vi "WSVCAP SHL Host LL RFFE Build and Parse Data.vi"(0 "Data Out":string, 1 "Data Out (Cycle Commands)":string[](array[string]), 2 "Post Command Delay":dbl[](array[numeric]) format="%#.0p s", 7 "Clock Rate (Hz) (Cycle Only)":dbl=50000.0, 9 "RFFE Data In [U8]":u8[][](array[numeric]) format="%02x", 12 "Simulate FPGA (Cycle Only)":bool, 13 "DUT Mask (All)":bool[](array[boolean])=[TRUE, TRUE, TRUE, TRUE, TRUE, TRUE, TRUE, TRUE, TRUE, TRUE, TRUE, TRUE, TRUE, TRUE, TRUE, TRUE, TRUE, TRUE, TRUE, TRUE, TRUE, TRUE, TRUE, TRUE, TRUE, TRUE, TRUE, TRUE, TRUE, TRUE, TRUE, TRUE, TRUE, TRUE, TRUE, TRUE]) -> (4 "RFFE Data Out [U8]":u8[][](array[numeric]) format="%02x", 6 "CMD Lengths (Bits)":u8[](array[numeric]), 8 "CMD Delays (Ticks)":u32[](array[numeric]), 10 "RFFE Data In":string[](array[string]))   [LabVIEW 2012]
panel:
  # "DUT 01"
  # "DUT 02"
  # "DUT 03"
  # "DUT 04"
  # "DUT 05"
  # "DUT 06"
  # "DUT 07"
  # "DUT 08"
  # "DUT 09"
  # "DUT 10"
  # "DUT 11"
  # "DUT 12"
  # "DUT 13"
  # "DUT 14"
  # "DUT 15"
  # "DUT 16"
  # "DUT 17"
  # "DUT 18"
  # "DUT 19"
  # "DUT 20"
  # "DUT 21"
  # "DUT 22"
  # "DUT 23"
  # "DUT 24"
  # "DUT 25"
  # "DUT 26"
  # "DUT 27"
  # "DUT 28"
  # "DUT 29"
  # "DUT 30"
  # "DUT 31"
  # "DUT 32"
  # "DUT 33"
  # "DUT 34"
  # "DUT 35"
  # "DUT 36"
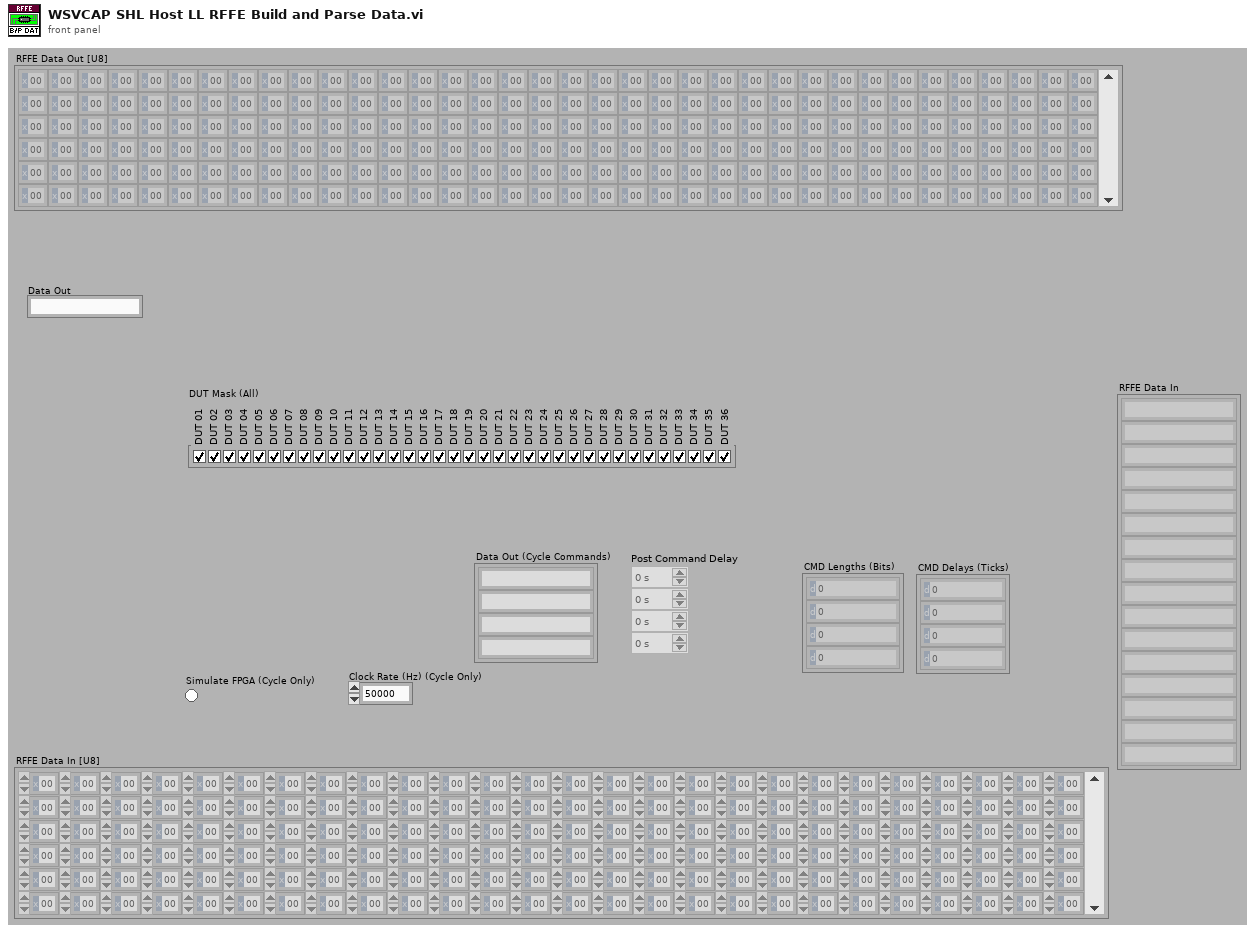
[diagram p1: front panel]
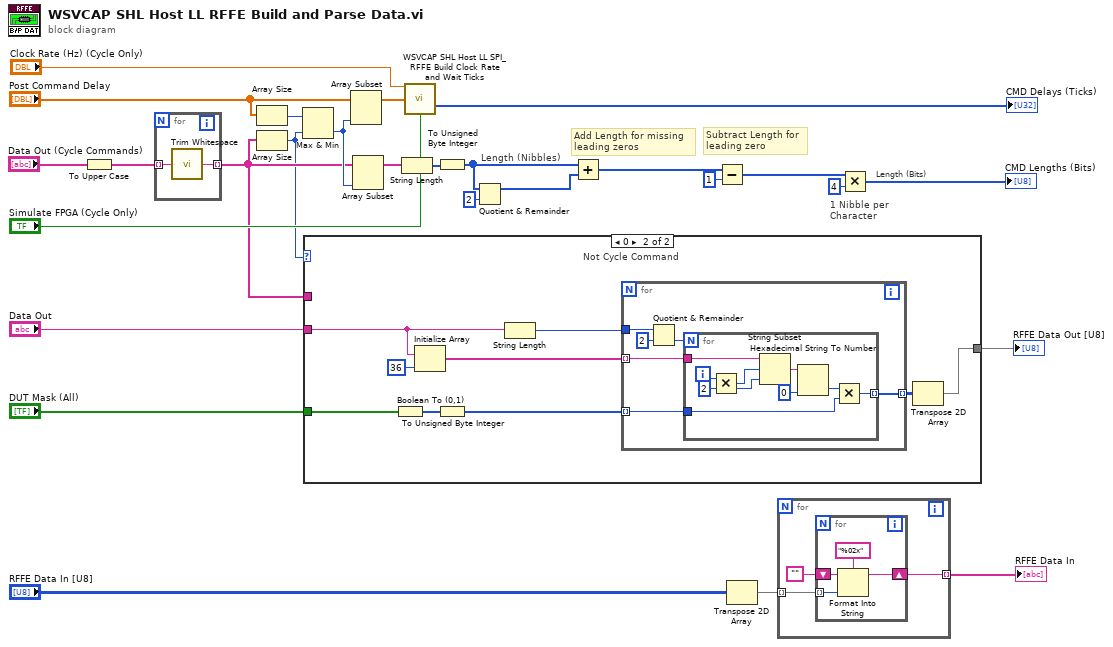
[diagram p0: block diagram]
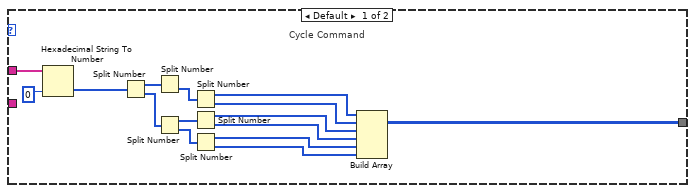
[diagram p2: hidden frame]
diagram:
  # "Subtract Length for\nleading zero"
  # "Add Length for missing\nleading zeros"
  # "Length (Bits)"
  # "Length (Nibbles)"
  # "1 Nibble per Character"
  n1 = To Upper Case(1:"Data Out (Cycle Commands)") -> (0:w1:string[])
  n2 = for {
    tunnel: w1 -> [w29] mode=indexing
    tunnel: [w28] -> w12 mode=indexing
    n3 = call <vilib>:"Trim Whitespace.vi"("string"=w29) -> ("trimmed string"=w28:string)  [unwired: 1 in]
  }
  n4 = Array Size(array="Post Command Delay") -> (size(s)=w21:i32)
  n5 = Array Size(array=w12) -> (size(s)=w11:i32)
  n6 = Max & Min(x=w21, y=w11) -> (min(x,y)=w18:i32)  [unwired: 1 out]
  n7 = case shown="0" w11 {
    tunnel: "DUT Mask (All)" -> [_ w53]
    tunnel: [w36 w48] -> w24
    tunnel: "Data Out" -> [_ w46]
    tunnel: w12 -> [w44 _]
    frame Default {
      # "Cycle Command"
      n8 = Hexadecimal String To Number(string=w44, default (0uL)=u64 0 ("Read Data")) -> (number=w37:u64[])  [unwired: 1 in, 1 out]
      n9 = Split Number(x=w37) -> (hi(x)=w42:u32[], lo(x)=w41:u32[])
      n10 = Split Number(x=w42) -> (lo(x)=w40:u16[])  [unwired: 1 out]
      n11 = Split Number(x=w41) -> (hi(x)=w39:u16[], lo(x)=w38:u16[])
      n12 = Split Number(x=w40) -> (hi(x)=w30:u8[], lo(x)=w35:u8[])
      n13 = Split Number(x=w39) -> (hi(x)=w34:u8[], lo(x)=w33:u8[])
      n14 = Split Number(x=w38) -> (hi(x)=w32:u8[], lo(x)=w31:u8[])
      n15 = Build Array(w30, w35, w34, w33, w32, w31) -> (w36:u8[][])
    }
    frame 0 {
      # "Not Cycle Command"
      n16 = Boolean To (0,1)(Boolean=w53) -> (0, 1=w52:i16[])
      n17 = Initialize Array(w46, 36 ("dimension size")) -> (w47:string[])
      n18 = To Unsigned Byte Integer(number=w52) -> (unsigned 8bit integer=w51:u8[])
      n19 = String Length(string=w46) -> (length=w45:i32)
      n20 = for {
        tunnel: w51 -> [w57] mode=indexing
        tunnel: [w56] -> w50 mode=indexing
        tunnel: w47 -> [w55] mode=indexing
        tunnel: w45 -> [w54]
        n21 = Quotient & Remainder(x=w54, y=2) -> (floor(x/y)=w58:i32)  [unwired: 1 out]
        n22 = for {
          N: w58 -> [_]
          tunnel: w55 -> [w68]
          tunnel: [w61] -> w56 mode=indexing
          tunnel: w57 -> [w62]
          i -> [w67]
          w65 = 2 ("y")
          n23 = Multiply(x=w67, y=w65) -> (x*y=w66:i32)
          n24 = String Subset(string=w68, offset (0)=w66, length (rest)=w65) -> (substring=w64:string)
          n25 = Hexadecimal String To Number(string=w64, default (0uL)=u8 0 ("default (0 U32)")) -> (number=w60:u8)  [unwired: 1 in, 1 out]
          n26 = Multiply(x=w60, y=w62) -> (x*y=w61:u8)
        }
      }
      n27 = Transpose 2D Array(2D array=w50) -> (transposed array=w48:u8[][])
    }
  }
  "RFFE Data Out [U8]" <- w24
  n28 = Array Subset(array="Post Command Delay", length=w18) -> (w19:dbl[])  [unwired: 1 in]
  n29 = Array Subset(array=w12, length=w18) -> (w17:string[])  [unwired: 1 in]
  n30 = String Length(string=w17) -> (length=w23:i32[])
  n31 = call "WSVCAP SHL Host LL SPI_RFFE Build Clock Rate and Wait Ticks.vi"("Clock Rate (Hz)"="Clock Rate (Hz) (Cycle Only)", "CMD Delay (s)"=w19, "Simulate FPGA"="Simulate FPGA (Cycle Only)") -> ("CMD Delay (Ticks)"=→"CMD Delays (Ticks)":u32[])  [unwired: 9 in, 3 out]
  n32 = To Unsigned Byte Integer(number=w23) -> (unsigned 8bit integer=w8:u8[])
  n33 = Quotient & Remainder(x=w8, y=u8 2) -> (x-y*floor(x/y)=w7:u8[])  [unwired: 1 out]
  n34 = Add(x=w8, y=w7) -> (x+y=w5:u8[])
  n35 = Subtract(x=w5, y=u8 1 ("Read Data")) -> (x-y=w3:u8[])
  n36 = Transpose 2D Array(2D array="RFFE Data In [U8]") -> (transposed array=w26:u8[][])
  n37 = for {
    tunnel: w26 -> [w71] mode=indexing
    tunnel: [w69] -> w25 mode=indexing
    n38 = for {
      tunnel: w71 -> [w75] mode=indexing
      shift-right: [w73] -> w69
      shift-left: "" -> [w72]
      n39 = Format Into String(format string="%02x", initial string=w72, w75) -> (resulting string=w73:string)  [unwired: 1 in, 1 out]
    }
  }
  "RFFE Data In" <- w25
  n40 = Multiply(x=w3, y=u8 4 ("Read Data")) -> (x*y=→"CMD Lengths (Bits)":u8[])
